vi "Adjust Dashboard Window.vi"(6 "Sizing Refnums":T1, 9 "Size Constraints":cluster{"min tab width":i32, "w/h":dbl}, 10 "VI":refnum<vi>, 11 "Notifier in":refnum<notifier>) -> ()   [LabVIEW 2014]
uses:
  <vilib>/Utility/miscctls.llb/LVRectTypeDef.ctl
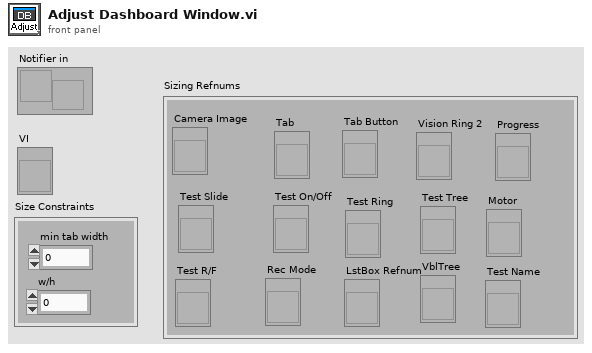
[diagram p1: front panel]
types:
  T1 = cluster{"Camera Image":refnum<vi>, "Tab":refnum<vi>, "Tab Button":refnum<vi>, "Vision Ring 2":refnum<vi>, "Rec Mode":refnum<vi>, "Test Slide":refnum<vi>, "Test On/Off":refnum<vi>, "Test Ring":refnum<vi>, "Test R/F":refnum<vi>, "Test Name":refnum<vi>, "Motor":refnum<vi>, "Progress":refnum<vi>, "LstBox Refnum":refnum<vi>, "Test Tree":refnum<vi>, "VblTree":refnum<vi>}
  T2 = typedef "LVRectTypeDef.ctl" = cluster{"Left":i16, "Top":i16, "Right":i16, "Bottom":i16}
  T3 = typedef "LVPointTypeDef.ctl" = cluster{"Horizontal":i16, "Vertical":i16}
  T4 = enum32{"Bad", "Idle", "Run top level", "Running"}
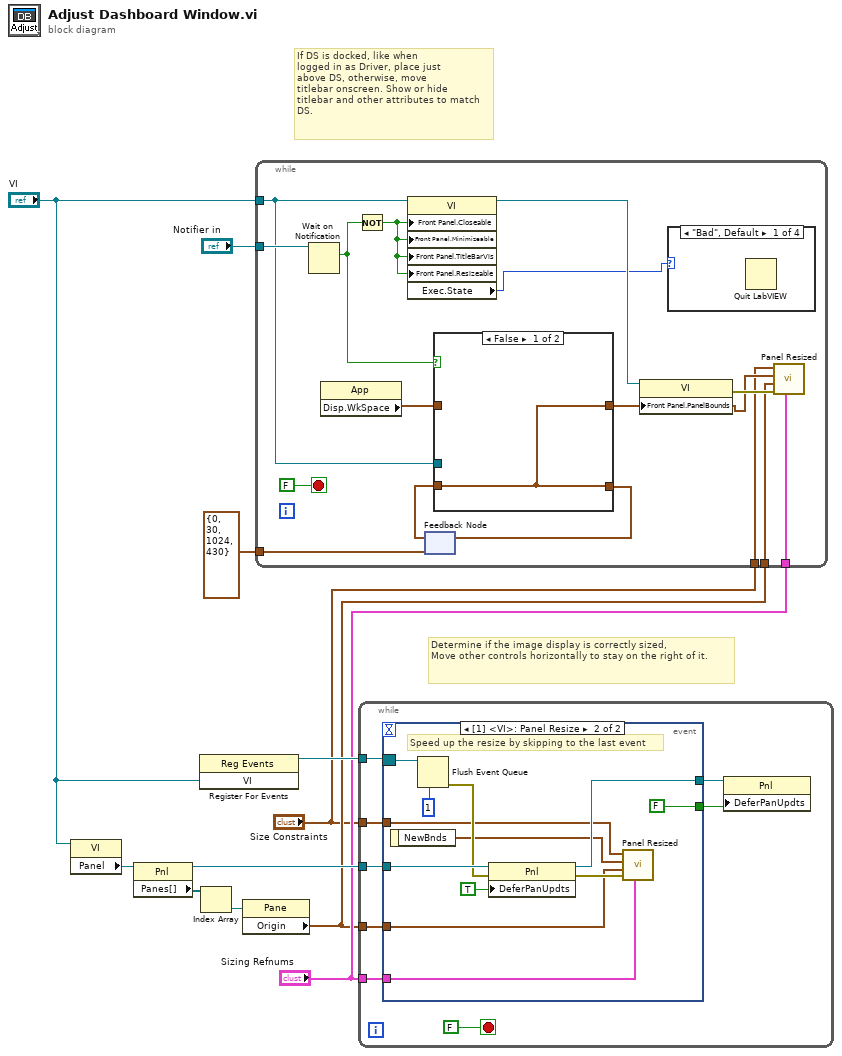
[diagram p0: block diagram]
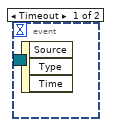
[diagram p2: hidden frame]
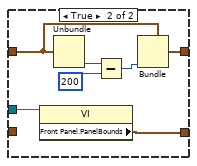
[diagram p6: hidden frame]
diagram:
  # "Determine if the image display is correctly sized,\nMove other controls horizontally to stay on the right of it."
  # "If DS is docked, like when\nlogged in as Driver, place just\nabove DS, otherwise, move\ntitlebar onscreen. Show or hide\ntitlebar and other attributes to match\nDS."
  n1 = property class="VI"(reference="VI") -> ("Panel"=w8:refnum<vi>)  [unwired: 1 in, 2 out]
  n2 = property class="Pnl"(reference=w8) -> (reference out=w5:refnum<vi>, "Panes[]"=w7:refnum<vi>[])  [unwired: 1 in, 1 out]
  n3 = register-events("VI") -> (reference out=w10:refnum<event-registration>)  [unwired: 2 in, 1 out]
  n4 = Index Array(array=w7) -> (element=w6:refnum<vi>)  [unwired: 1 in]
  n5 = property class="Pane"(reference=w6) -> ("Origin"=w3:T3)  [unwired: 1 in, 2 out]
  n6 = while {
    tunnel: "Notifier in" -> [w26]
    tunnel: "VI" -> [w17]
    tunnel: "Sizing Refnums" -> [w22]
    tunnel: w3 -> [w21]
    tunnel: "Size Constraints" -> [w19]
    tunnel: T2 {"Left"=0, "Top"=30, "Right"=1024, "Bottom"=430} ("Front Panel.PanelBounds") -> [w14]
    stop <- FALSE stop-if-true
    n7 = Wait on Notification(notifier=w26) -> (notification=w18:bool)  [unwired: 3 in, 3 out]
    n8 = property class="App"() -> ("Disp.WkSpace"=w25:T2)  [unwired: 2 in, 2 out]
    n9 = Not(x=w18) -> (.not. x?=w13:bool)
    n10 = property class="VI"(reference=w17, "Front Panel.Closeable"=w13, "Front Panel.Minimizeable"=w13, "Front Panel.TitleBarVis"=w13, "Front Panel.Resizeable"=w13) -> (reference out=w24:refnum<vi>, "Exec.State"=w12:T4)  [unwired: 1 in, 1 out]
    n11 = feedback #1(w14) -> (w15:T2)
    n12 = case shown="False" w18 {
      tunnel: w25 -> [_ w31]
      tunnel: [w28 w32] -> w20
      tunnel: w17 -> [_ w30]
      tunnel: [w28 w29] -> w16
      tunnel: w15 -> [w28 _]
      frame False {
      }
      frame True {
        n13 = property class="VI"(reference=w30) -> ("Front Panel.PanelBounds"=w29:T2)  [unwired: 1 in, 2 out]
        n14 = Unbundle(w31) -> ("Bottom"=w35:i16)  [unwired: 3 out]
        n15 = Subtract(x=w35, y=200) -> (x-y=w33:i32)
        n16 = Bundle(cluster=w31, "Bottom"=w33) -> (w32:T2)  [unwired: 3 out]
      }
    }
    n17 = feedback-in #1(w16) -> ()
    n18 = property class="VI"(reference=w24, "Front Panel.PanelBounds"=w20) -> (error out=w23:errorcluster)  [unwired: 1 in, 1 out]
    n19 = case shown="\"Bad\", Default" w12 {
      frame "Bad", Default {
        n20 = Quit LabVIEW() -> ()  [unwired: 1 in]
      }
      frame "Idle" {
      }
      frame "Run top level" {
      }
      frame "Running" {
      }
    }
    n21 = call "Panel Resized.vi"("Sizing Refnums"=w22, "error in (no error)"=w23, "Origin"=w21, "NewBnds"=w20, "Size Constraints"=w19) -> ()  [unwired: 6 in, 1 out]
  }
  n22 = while {
    tunnel: w10 -> [w42]
    tunnel: "Sizing Refnums" -> [w41]
    tunnel: "Size Constraints" -> [w40]
    tunnel: w3 -> [w39]
    tunnel: w5 -> [w38]
    stop <- FALSE stop-if-true
    n23 = event shown="[1] <VI>: Panel Resize" {
      selector: w42 -> [_ w52]
      dyn-events: _ -> [_ _]
      timeout: _ -> [_ _]
      tunnel: w41 -> [_ w44]
      tunnel: w40 -> [_ w47]
      tunnel: w39 -> [_ w45]
      tunnel: w38 -> [_ w55]
      tunnel: [_ FALSE ("Defer Panel Updates")] -> w37
      tunnel: [_ w49] -> w36
      event Timeout {
        n24 = event-data() -> ()  [unwired: 1 in, 3 out]
      }
      event Panel Resize {
        # "Speed up the resize by skipping to the last event"
        n25 = event-data() -> ("NewBnds"=w46:T2)  [unwired: 1 in]
        n26 = Flush Event Queue(0:w52, 5:1 ("keep most recent")) -> (11:w50:errorcluster)  [unwired: 4 in, 2 out]
        n27 = property class="Pnl"(reference=w55, error in=w50, "DeferPanUpdts"=TRUE ("Defer Panel Updates")) -> (reference out=w49:refnum<vi>, error out=w48:errorcluster)
        n28 = call "Panel Resized.vi"("Sizing Refnums"=w44, "error in (no error)"=w48, "Origin"=w45, "NewBnds"=w46, "Size Constraints"=w47) -> ()  [unwired: 6 in, 1 out]
      }
    }
    n29 = property class="Pnl"(reference=w36, "DeferPanUpdts"=w37) -> ()  [unwired: 1 in, 2 out]
  }
